vi "Enable Process.vi"(8 "Error In":errorcluster, 9 "Run?":bool=TRUE, 10 "Process Name":string, 11 "CS++DSCManager in":refnum<class "CS++DSCManager.lvclass">) -> (0 "Error Out":errorcluster, 3 "CS++DSCManager out":refnum<class "CS++DSCManager.lvclass">)   [LabVIEW 2014, in "CS++DSCManager.lvlib" / "CS++DSCManager.lvclass"]
doc: "Toggles the run state of a process in the Shared Variable Engine."
uses:
  CS++DSCManager.lvclass
  <vilib>/lvdsc/NI_DSC.lvlib
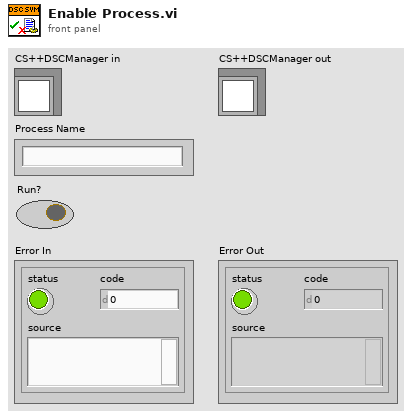
[diagram p1: front panel]
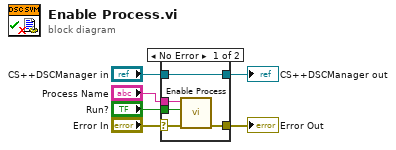
[diagram p0: block diagram]
diagram:
  n1 = case shown="No Error" "Error In" {
    selector: "Error In" -> [w10 w13]
    tunnel: [w9 w13] -> w5
    tunnel: [w11 w12] -> w3
    tunnel: "CS++DSCManager in" -> [w11 w12]
    tunnel: "Process Name" -> [w8 _]
    tunnel: "Run?" -> [w7 _]
    frame No Error {
      n2 = call <vilib>:"Enable Process.vi"("error in (no error)"=w10, "run?"=w7, "process name"=w8) -> ("error out"=w9:errorcluster)  [unwired: 7 in, 1 out]
    }
    frame Error {
    }
  }
  "Error Out" <- w5
  "CS++DSCManager out" <- w3
